vi "rvc SIM Control Mixer.vi"(8 "T":dbl, 9 "tau yaw":dbl, 10 "tau roll":dbl, 11 "tau pitch":dbl) -> (0 "w4":dbl, 1 "w3":dbl, 2 "w2":dbl, 3 "w1":dbl)   [LabVIEW 2013]
uses:
  <vilib>/Simulation/Implementation/Shared/SIMSCR Execution Mode.ctl
  <vilib>/Simulation/Scripting/Companion Diagram/SimConfigNode/SimParams.ctl
  <vilib>/Simulation/Scripting/Companion Diagram/SimConfigNode/_simSolvers.ctl
  <vilib>/Simulation/Param Hierarchy/Typedefs/SIMPH Param Control Actions.ctl
  <vilib>/Simulation/Implementation/Shared/NILVSim_ParamChanged.vi
  <vilib>/Simulation/Implementation/Shared/NILVSIM_BeginStep.vi
  <vilib>/Simulation/Nonlinear/Implementation/NILVSim Saturation.llb/SIM Saturation (scalar).vi
  <vilib>/Simulation/SignalArithmetic/Implementation/NILVSim Gain.llb/SIM Gain (scalar).vi
  <vilib>/Simulation/Implementation/Shared/NILVSim_Manager.vi
  <vilib>/Simulation/Implementation/Shared/NILVSim_FinalizeModel.vi
  <vilib>/Simulation/Implementation/Shared/SIM Unbundle Sim Info.vi
  <vilib>/Utility/error.llb/Clear Errors.vi
  <vilib>/Simulation/Implementation/Shared/NILVSim_GetModelError.vi
  <vilib>/Simulation/Implementation/Shared/SIM SimErrorHandler.vi
  <vilib>/Simulation/Implementation/Shared/SIM Bundle Sim Info.vi
  <vilib>/Simulation/Implementation/Shared/SIMSH Read Queue.vi
  <vilib>/Simulation/Implementation/Shared/NILVSim_Initialize.vi
  <vilib>/Simulation/Utility/Implementation/NILVSim Get Time and IsAcceptedStep.vi
  <vilib>/Simulation/Scripting/Companion Diagram/SimConfigNode/SimDog.xnode
  <vilib>/Simulation/Implementation/XNodeFramework/SimXNode/SimX.xnode
  <vilib>/Simulation/Implementation/Shared/NI_SIM_Implementation.lvlib
panel:
  out "all":dbl[](array[numeric])
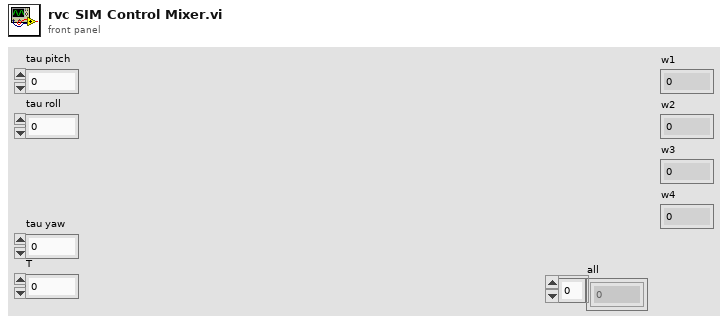
[diagram p1: front panel]
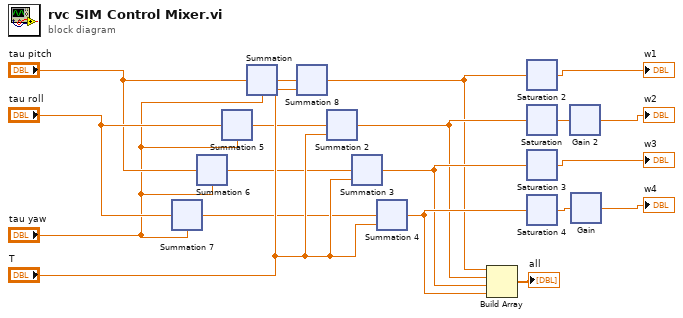
[diagram p0: block diagram]
diagram:
  n1 = xnode ("Summation 7")("Operand1"="tau roll", "Operand2"="tau yaw") -> ("Result"=w11:dbl)
  n2 = xnode ("Summation 6")("Operand1"="tau pitch", "Operand2"="tau yaw") -> ("Result"=w10:dbl)
  n3 = xnode ("Summation 5")("Operand1"="tau roll", "Operand2"="tau yaw") -> ("Result"=w9:dbl)
  n4 = xnode ("Summation")("Operand1"="tau pitch", "Operand2"="tau yaw") -> ("Result"=w8:dbl)
  n5 = xnode ("Summation 8")("Operand1"=w8, "Operand2"="T") -> ("Result"=w12:dbl)
  n6 = xnode ("Summation 2")("Operand1"=w9, "Operand2"="T") -> ("Result"=w13:dbl)
  n7 = xnode ("Summation 3")("Operand1"=w10, "Operand2"="T") -> ("Result"=w14:dbl)
  n8 = xnode ("Summation 4")("Operand1"=w11, "Operand2"="T") -> ("Result"=w15:dbl)
  n9 = Build Array(w12, w13, w14, w15) -> (→"all":dbl[])
  n10 = xnode ("Saturation 2")("input"=w12) -> ("output"=→"w1":dbl)  [unwired: 4 in]
  n11 = xnode ("Saturation")("input"=w13) -> ("output"=w4:dbl)  [unwired: 4 in]
  n12 = xnode ("Saturation 3")("input"=w14) -> ("output"=→"w3":dbl)  [unwired: 4 in]
  n13 = xnode ("Saturation 4")("input"=w15) -> ("output"=w6:dbl)  [unwired: 4 in]
  n14 = xnode ("Gain 2")("input"=w4) -> ("output"=→"w2":dbl)  [unwired: 3 in]
  n15 = xnode ("Gain")("input"=w6) -> ("output"=→"w4":dbl)  [unwired: 3 in]
